vi "Vision Research Phantom Series PhFile PhEnableCine16Bpp.vi"(0 "Simulate? (False)":bool, 1 "CH in":u32, 3 "bEnable16Bpp":u32, 5 "Error In (no error)":errorcluster) -> (15 "CH out":u32=1, 19 "Error Out":errorcluster)   [LabVIEW 2013, in "VRI.lvlib"]
doc: "PhFile.dll\n\nPhEnableCine16Bpp\nEXIMPROC HRESULT PhEnableCine16Bpp(CINEHANDLE CH, BOOL bEnable16Bpp);\n\nParameters Description\nCH(in) Handle of the cine to be saved.\nbEnable16Bpp(in) TRUE to activate 16 bpp image format for the cine\n FALSE to deactivate it\nReturn HRESULT (0 = Ok)\n ERR_BadCine - Cine handle was not initialized. \nComments Activates/Deactivates 16bpp image format for Phantom camera cines.\n The operation changes the cine's BITMAPINFOHEADER. \n Call PhGetCineBMIH to get the new BITMAPINFOHEADER."
uses:
  VRI.lvlib
  Projects/SDK/32-bit/Vision Research Phantom Series Labview Driver/Phantom DLLs/PhFile.dll
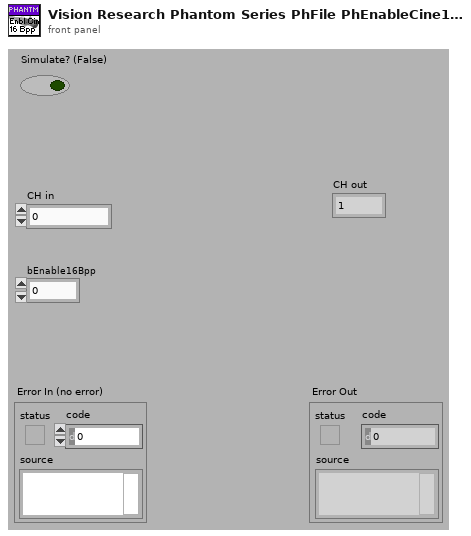
[diagram p1: front panel]
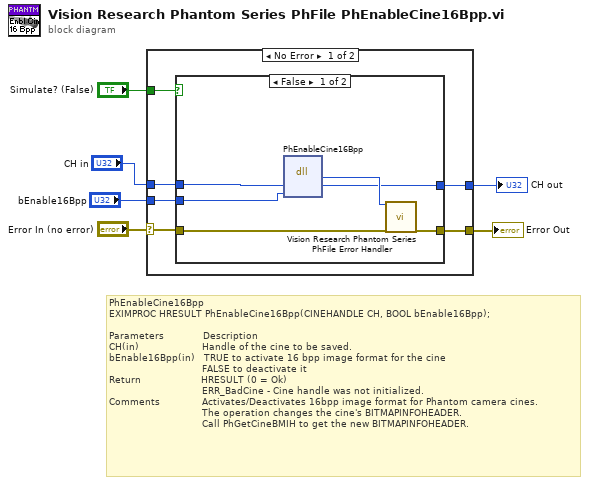
[diagram p0: block diagram]
diagram:
  # "PhEnableCine16Bpp\nEXIMPROC HRESULT PhEnableCine16Bpp(CINEHANDLE CH, BOOL bEnable16Bpp);\n\nParameters             Description\nCH(in)                     Handle of the cine to be saved.\nbEnable16Bpp(in)   TRUE to activate 16 bpp image format for the cine\n                               FALSE to deactivate it\nReturn                    HRESULT (0 = Ok)\n                               ERR_BadCine - Cine handle was not initialized. \nComments              Activates/Deactivates 16bpp image format for Phantom camera cines.\n                               The operation changes the cine's BITMAPINFOHEADER. \n                               Call PhGetCineBMIH to get the new BITMAPINFOHEADER."
  n1 = case shown="No Error" "Error In (no error)" {
    selector: "Error In (no error)" -> [w12 w22]
    tunnel: [w11 w22] -> w5
    tunnel: "Simulate? (False)" -> [w10 _]
    tunnel: "CH in" -> [w9 w21]
    tunnel: "bEnable16Bpp" -> [w8 _]
    tunnel: [w7 w21] -> w1
    frame No Error {
      n2 = case shown="False" w10 {
        tunnel: w12 -> [w17 w20]
        tunnel: [w18 w20] -> w11
        tunnel: w9 -> [w16 w19]
        tunnel: w8 -> [w14 _]
        tunnel: [w13 w19] -> w7
        frame False {
          n3 = dll-call lib="C:/Projects/SDK/32-bit/Vision Research Phantom Series Labview Driver/Phantom DLLs/PhFile.dll" fn="PhEnableCine16Bpp"("CH"=w16, "bEnable16Bpp"=w14) -> ("HRESULT"=w15:i32, "CH"=w13:u32)  [unwired: 4 in, 2 out]
          n4 = call "Vision Research Phantom Series PhFile Error Handler.vi"("Error Code (0)"=w15, "Error In (no error)"=w17) -> ("Error Out"=w18:errorcluster)  [unwired: 17 out]
        }
        frame True {
          # "It looks as though the dlls can provide simulated data so this case may not have to be used"
        }
      }
    }
    frame Error {
    }
  }
  "Error Out" <- w5
  "CH out" <- w1
